vi "OAT Overall Level Plot.vi"   [LabVIEW 2017, in "SoundVib_OrderTracking.lvlib"]
doc: "Computes the root-mean-square (RMS) level of the <B>even-angle signal</B> and generates an XY graph as the output. Wire data to the <B>even-angle signal</B> input to determine the polymorphic instance to use or manually select the instance."
uses:
  <vilib>/addons/Sound and Vibration/Order Analysis/Resample Order Tracking/SoundVib_OrderTracking.lvlib
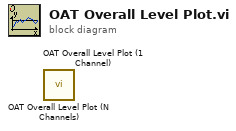
[diagram p0: block diagram]
diagram:
  n1 = call <vilib>:"OAT Overall Level Plot (N Channels).vi"() -> ()  [unwired: 12 in, 4 out]
  n2 = call <vilib>:"OAT Overall Level Plot (1 Channel).vi"() -> ()  [unwired: 12 in, 4 out]
